vi "AppendToOutput.vi"(3 "error in":errorcluster, 4 "Input String":string, 5 "Output Refnum In":refnum<vi>) -> (0 "error out":errorcluster, 2 "Output Refnum Out":refnum<vi>)   [LabVIEW 2013]
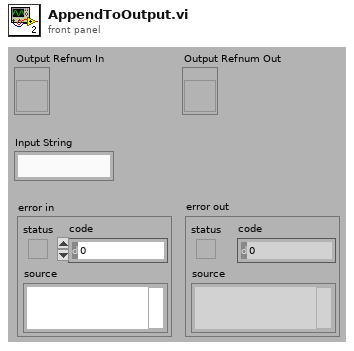
[diagram p1: front panel]
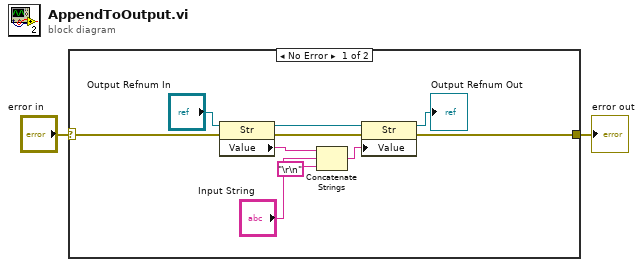
[diagram p0: block diagram]
diagram:
  n1 = case shown="No Error" "error in" {
    selector: "error in" -> [w3 w13]
    tunnel: [w4 w13] -> w2
    frame No Error {
      n2 = property on="Property Node" class="Str"(reference="Output Refnum In", error in=w3) -> (reference out=w6:refnum<vi>, error out=w5:errorcluster, "Value"=w10:string)
      n3 = Concatenate Strings(w10, "Input String", "\r\n") -> (w9:string)
      n4 = property class="Str"(reference=w6, error in=w5, "Value"=w9) -> (reference out=→"Output Refnum Out":refnum<vi>, error out=w4:errorcluster)
    }
    frame Error {
    }
  }
  "error out" <- w2
